vi "Save Sweep Settings File.vi"(7 "Seq File Ref In":refnum<k7>, 8 "error in (no error)":errorcluster, 10 "Sweep Settings Data":T1[](array[typedef]) {"Sweep Points"."Frequency" format="%#_6p"}, 11 "New Sequence File Path":path) -> (0 "error out":errorcluster, 5 "Seq File Ref Out":refnum<k7>)   [LabVIEW 2016]
uses:
  RFPM CLB Calibration/RFPM CLB Calibration UI.lvlibp/Actors/RFPM CLB Calibration Process/RFPM CLB Calibration Process/TypeDefs/Sweep Type.ctl
  RFPM CLB Calibration/RFPM CLB Calibration UI.lvlibp/Actors/RFPM CLB Calibration Process/RFPM CLB Calibration Process/TypeDefs/Sweep Settings.ctl
  RFPM CLB Calibration/RFPM CLB Calibration UI.lvlibp/Actors/RFPM CLB Calibration UI/RFPM CLB Calibration UI/TypeDefs/Sweep Points.ctl
  RFPM CLB Calibration/RFPM CLB Calibration UI.lvlibp/Actors/RFPM CLB Calibration UI/RFPM CLB Calibration UI/TypeDefs/Sweep Editor Data.ctl
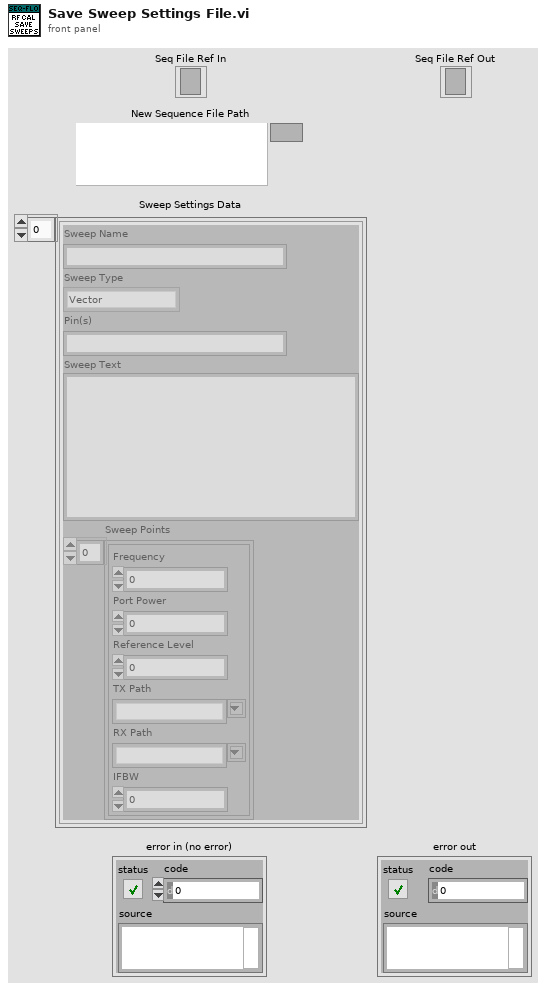
[diagram p1: front panel]
types:
  T1 = typedef "RFPM CLB Calibration UI.lvlibp/RFPM CLB Calibration UI.lvclass/Sweep Editor Data.ctl" = cluster{"Sweep Name":string, "Sweep Type":T2, "Pin(s)":string, "Sweep Text":string, "Sweep Points":T3[]}
  T2 = typedef "RFPM CLB Calibration UI.lvlibp/RFPM CLB Calibration Process.lvlib/RFPM CLB Calibration Process.lvclass/Sweep Type.ctl" = enum16{"Vector", "Source", "Receiver"}
  T3 = typedef "RFPM CLB Calibration UI.lvlibp/RFPM CLB Calibration UI.lvclass/Sweep Points.ctl" = cluster{"Frequency":dbl, "Port Power":dbl, "Reference Level":dbl, "TX Path":string, "RX Path":string, "IFBW":dbl}
  T4 = typedef "RFPM CLB Calibration UI.lvlibp/RFPM CLB Calibration Process.lvlib/RFPM CLB Calibration Process.lvclass/Sweep Settings.ctl" = cluster{"Sweep Name":string, "Sweep Type":T2, "Pins":string[]}
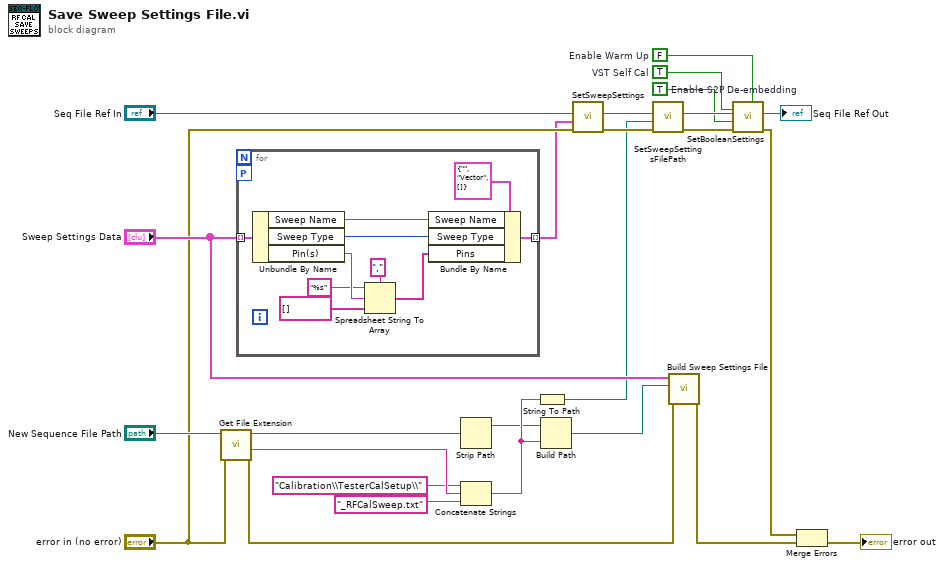
[diagram p0: block diagram]
diagram:
  w10 = FALSE  # Enable Warm Up
  w11 = TRUE  # VST Self Cal
  w12 = TRUE  # Enable S2P De-embedding
  n1 = call <vilib>:"Get File Extension.vi"("error in (no error)"="error in (no error)", "file"="New Sequence File Path") -> ("error out"=w23:errorcluster, "filename without extension"=w22:string, "dup file"=w24:path)  [unwired: 5 in, 2 out]
  n2 = for {
    tunnel: "Sweep Settings Data" -> [w35] mode=indexing
    tunnel: [w32] -> w1 mode=indexing
    workers-P: _ -> [_]
    n3 = Unbundle By Name(w35) -> ("Sweep Name"=w33:string, "Sweep Type"=w34:T2, "Pin(s)"=w31:string)
    n4 = Spreadsheet String To Array(delimiter (Tab)=",", format string="%s", spreadsheet string=w31, array type (2D Dbl)=string[] []) -> (array=w28:string[])
    n5 = Bundle By Name(cluster=T4 {"Sweep Name"="", "Sweep Type"=enum."Vector", "Pins"=[]}, "Sweep Name"=w33, "Sweep Type"=w34, "Pins"=w28) -> (w32:T4)
  }
  n6 = Strip Path(path=w24) -> (stripped path=w4:path)  [unwired: 1 out]
  n7 = Concatenate Strings("Calibration\\TesterCalSetup\\" ("string"), w22, "_RFCalSweep.txt" ("string")) -> (w6:string)
  n8 = String To Path(string=w6) -> (path=w3:path)
  n9 = Build Path(base path=w4, name or relative path=w6) -> (appended path=w5:path)
  n10 = call "SetSweepSettings.vi"("error in (no error)"="error in (no error)", "Sweep Settings"=w1, "Seq File Ref In"="Seq File Ref In") -> ("error out"=w20:errorcluster, "Seq File Ref Out"=w17:refnum<k7>)  [unwired: 6 in, 1 out]
  n11 = call "SetSweepSettingsFilePath.vi"("error in (no error)"=w20, "Sweep Settings File Path"=w3, "Seq File Ref In"=w17) -> ("error out"=w9:errorcluster, "Seq File Ref Out"=w13:refnum<k7>)  [unwired: 6 in, 1 out]
  n12 = call "Build Sweep Settings File.vi"("error in"=w23, "Path"=w5, "Sweep Settings Data"="Sweep Settings Data") -> ("error out"=w15:errorcluster)  [unwired: 7 in, 1 out]
  n13 = call "SetBooleanSettings.vi"("Enable Warm Up"=w10, "VST Self Cal"=w11, "error in (no error)"=w9, "Enable S2P De-embedding"=w12, "Seq File Ref In"=w13) -> ("error out"=w8:errorcluster, "Seq File Ref Out"=→"Seq File Ref Out":refnum<k7>)  [unwired: 4 in, 1 out]
  n14 = Merge Errors(w8, w15) -> (→"error out":errorcluster)
